vi "cw_3_2.vi"() -> ()   [LabVIEW 2022 SP3]
panel:
  out "Array":i32[][](array[numeric])
  in  "M":i32
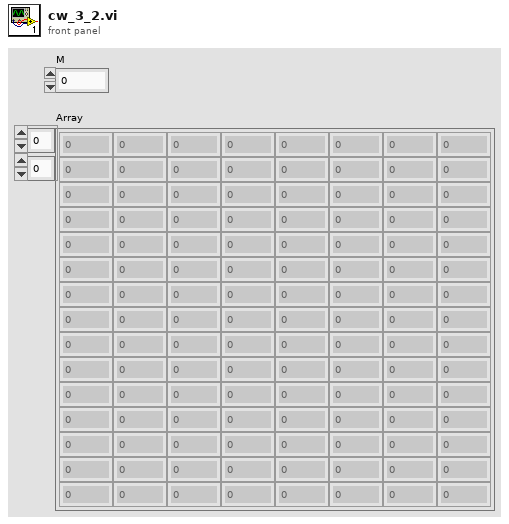
[diagram p1: front panel]
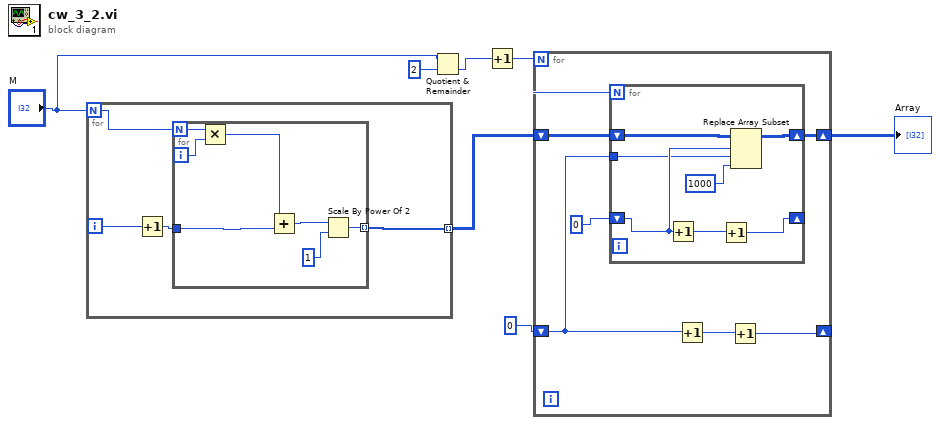
[diagram p0: block diagram]
diagram:
  n1 = for {
    N: "M" -> [w11]
    tunnel: [w10] -> w5 mode=indexing
    i -> [w9]
    n2 = Increment(x=w9) -> (x+1=w8:i32)
    n3 = for {
      N: w11 -> [w15]
      tunnel: [w18] -> w10 mode=indexing
      tunnel: w8 -> [w12]
      i -> [w16]
      n4 = Multiply(x=w15, y=w16) -> (x*y=w14:i32)
      n5 = Add(x=w14, y=w12) -> (x+y=w13:i32)
      n6 = Scale By Power Of 2(n=w13, x=1) -> (x*2^n=w18:i32)
    }
  }
  n7 = Quotient & Remainder(x="M", y=2) -> (floor(x/y)=w2:i32)  [unwired: 1 out]
  n8 = Increment(x=w2) -> (x+1=w1:i32)
  n9 = for {
    N: w1 -> [w25]
    shift-right: [w23] -> w4
    shift-left: w5 -> [w24]
    shift-right: [w20] -> _
    shift-left: 0 -> [w19]
    n10 = for {
      N: w25 -> [_]
      shift-right: [w31] -> w23
      shift-left: w24 -> [w32]
      shift-right: [w28] -> _
      shift-left: 0 -> [w27]
      tunnel: w19 -> [w26]
      n11 = Increment(x=w27) -> (x+1=w29:i32)
      n12 = Increment(x=w29) -> (x+1=w28:i32)
      n13 = Replace Array Subset(array=w32, new element=1000 ("new element/subarray"), index (row)=w27, index (col)=w26) -> (w31:i32[][])
    }
    n14 = Increment(x=w19) -> (x+1=w21:i32)
    n15 = Increment(x=w21) -> (x+1=w20:i32)
  }
  "Array" <- w4
